vi "GT Add Event Task Link.vi"(7 "pLinkIndex":i16, 8 "error in (no error)":errorcluster caption="错误输入（无错误）", 9 "taskIndex":i16, 10 "eventIndex":i16, 11 "cardNum":i16) -> (0 "error out":errorcluster caption="错误输出", 3 "function return":i16, 5 "pLinkIndex out":i16)   [LabVIEW 2020, in "gts1.lvlib"]
doc: "GT_API GT_AddEventTaskLink(short cardNum,short eventIndex,short taskIndex,short *pLinkIndex);"
uses:
  gts1.lvlib
  dll/32bit/multi_card/gts.dll
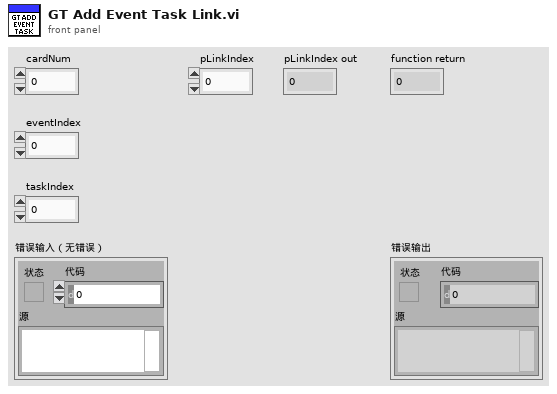
[diagram p1: front panel]
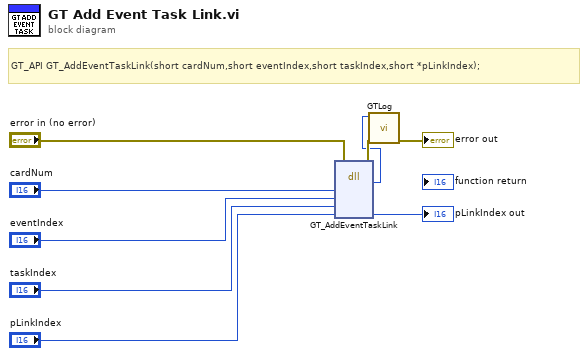
[diagram p0: block diagram]
diagram:
  # "GT_API GT_AddEventTaskLink(short cardNum,short eventIndex,short taskIndex,short *pLinkIndex);"
  n1 = dll-call lib="C:/1228/dll/32bit/multi_card/gts.dll" fn="GT_AddEventTaskLink"(error in="error in (no error)", "cardNum"="cardNum", "eventIndex"="eventIndex", "taskIndex"="taskIndex", "pLinkIndex"="pLinkIndex") -> (error out=w3:errorcluster, "return type"=w1:i16, "pLinkIndex"=→"pLinkIndex out":i16)  [unwired: 5 in, 1 out]
  n2 = call "GTLog.vi"("error in (no error)"=w3, "Numeric"=w1) -> ("error out"=→"error out":errorcluster)  [unwired: 9 in]
